vi "RTS Headers.vi"(4 "CSV Data Save Input":T1, 6 "Save Data":bool, 7 "All Data?":bool, 8 "Error In":errorcluster, 9 "RTS Config Setup Input":T3, 10 "Station":u8=1 min=1 max=8 step=1, 11 "Chamber 1 Data in":T12 {"Room PID Settings"."Room Dehumid Temperature I (*RM Dehum I1)" max=30000 step=1; "Room PID Settings"."Room Dehumid Temperature P (*RM Dehum P1)" max=30000 step=1; "Room PID Settings"."Room Cool Temperature I (*RM Cool I1)" max=30000 step=1; "Room PID Settings"."Room Cool Temperature P (*RM Cool P1)" max=30000 step=1; "Room PID Settings"."Room Heat I (*RM Heat I1)" max=30000 step=1; "Room PID Settings"."Room Heat P (*RM Heat P1)" max=30000 step=1; "Room PID Settings"."Room Humidity I (*RM Hum I1)" max=30000 step=1; "Room PID Settings"."Room Humidity P (*RM Hum P1)" max=30000 step=1; "Room PID Settings"."Room Dry I (*RM Dry I1)" max=30000 step=1; "Room PID Settings"."Room Dry P(*RM Dry P1)" max=30000 step=1; "Station 8"."Voltage (V):Element 1 Avg" format="%.3g"; "Station 8"."Voltage (V):Element 2 Avg" format="%.3g"; "Station 8"."Max Watt Hours" format="%.3g"; "Station 8"."Power Factor:Element 2" format="%.3g"; "Station 8"."Power Factor:Element 1" format="%.3g"; "Station 8"."Apparent Power (VA):Element 2" format="%.3g"; "Station 8"."Apparent Power (VA):Element 1" format="%.3g"; "Station 8"."Frequency (Hz):Element 1" format="%.3g"; "Station 8"."Time:Element 1" format="%.3g"; "Station 8"."Voltage Crest Factor:Element 2" format="%.3g"; "Station 8"."Voltage Crest Factor:Element 1" format="%.3g"; "Station 8"."Voltage Harmonic (%):Element 2" format="%.3g"; "Station 8"."Voltage Harmonic (%):Element 1" format="%.3g"; "Station 8"."Current Crest Factor:Element 2" format="%.3g"; "Station 8"."Current Crest Factor:Element 1" format="%.3g"; "Station 8"."Voltage (V):Element 1" format="%.3g"; "Station 8"."Voltage (V):Element 2" format="%.3g"; "Station 8"."Watt Hours (Wh):Sigma" format="%.3f"; "Station 8"."Power (W):Sigma" format="%.3g"; "Station 8"."Current (A):Element 2" format="%.3g"; "Station 8"."Current (A):Element 1" format="%.3g"; "Station 7"."Voltage (V):Element 1 Avg" format="%.3g"; "Station 7"."Voltage (V):Element 2 Avg" format="%.3g"; "Station 7"."Max Watt Hours" format="%.3g"; "Station 7"."Power Factor:Element 2" format="%.3g"; "Station 7"."Power Factor:Element 1" format="%.3g"; "Station 7"."Apparent Power (VA):Element 2" format="%.3g"; "Station 7"."Apparent Power (VA):Element 1" format="%.3g"; "Station 7"."Frequency (Hz):Element 1" format="%.3g"; "Station 7"."Time:Element 1" format="%.3g"; "Station 7"."Voltage Crest Factor:Element 2" format="%.3g"; "Station 7"."Voltage Crest Factor:Element 1" format="%.3g"; "Station 7"."Voltage Harmonic (%):Element 2" format="%.3g"; "Station 7"."Voltage Harmonic (%):Element 1" format="%.3g"; "Station 7"."Current Crest Factor:Element 2" format="%.3g"; "Station 7"."Current Crest Factor:Element 1" format="%.3g"; "Station 7"."Voltage (V):Element 1" format="%.3g"; "Station 7"."Voltage (V):Element 2" format="%.3g"; "Station 7"."Watt Hours (Wh):Sigma" format="%.3f"; "Station 7"."Power (W):Sigma" format="%.3g"; "Station 7"."Current (A):Element 2" format="%.3g"; "Station 7"."Current (A):Element 1" format="%.3g"; "Station 6"."Voltage (V):Element 1 Avg" format="%.3g"; "Station 6"."Voltage (V):Element 2 Avg" format="%.3g"; "Station 6"."Max Watt Hours" format="%.3g"; "Station 6"."Power Factor:Element 2" format="%.3g"; "Station 6"."Power Factor:Element 1" format="%.3g"; "Station 6"."Apparent Power (VA):Element 2" format="%.3g"; "Station 6"."Apparent Power (VA):Element 1" format="%.3g"; "Station 6"."Frequency (Hz):Element 1" format="%.3g"; "Station 6"."Time:Element 1" format="%.3g"; "Station 6"."Voltage Crest Factor:Element 2" format="%.3g"; "Station 6"."Voltage Crest Factor:Element 1" format="%.3g"; "Station 6"."Voltage Harmonic (%):Element 2" format="%.3g"; "Station 6"."Voltage Harmonic (%):Element 1" format="%.3g"; "Station 6"."Current Crest Factor:Element 2" format="%.3g"; "Station 6"."Current Crest Factor:Element 1" format="%.3g"; "Station 6"."Voltage (V):Element 1" format="%.3g"; "Station 6"."Voltage (V):Element 2" format="%.3g"; "Station 6"."Watt Hours (Wh):Sigma" format="%.3f"; "Station 6"."Power (W):Sigma" format="%.3g"; "Station 6"."Current (A):Element 2" format="%.3g"; "Station 6"."Current (A):Element 1" format="%.3g"; "Station 5"."Voltage (V):Element 1 Avg" format="%.3g"; "Station 5"."Voltage (V):Element 2 Avg" format="%.3g"; "Station 5"."Max Watt Hours" format="%.3g"; "Station 5"."Power Factor:Element 2" format="%.3g"; "Station 5"."Power Factor:Element 1" format="%.3g"; "Station 5"."Apparent Power (VA):Element 2" format="%.3g"; "Station 5"."Apparent Power (VA):Element 1" format="%.3g"; "Station 5"."Frequency (Hz):Element 1" format="%.3g"; "Station 5"."Time:Element 1" format="%.3g"; "Station 5"."Voltage Crest Factor:Element 2" format="%.3g"; "Station 5"."Voltage Crest Factor:Element 1" format="%.3g"; "Station 5"."Voltage Harmonic (%):Element 2" format="%.3g"; "Station 5"."Voltage Harmonic (%):Element 1" format="%.3g"; "Station 5"."Current Crest Factor:Element 2" format="%.3g"; "Station 5"."Current Crest Factor:Element 1" format="%.3g"; "Station 5"."Voltage (V):Element 1" format="%.3g"; "Station 5"."Voltage (V):Element 2" format="%.3g"; "Station 5"."Watt Hours (Wh):Sigma" format="%.3f"; "Station 5"."Power (W):Sigma" format="%.3g"; "Station 5"."Current (A):Element 2" format="%.3g"; "Station 5"."Current (A):Element 1" format="%.3g"; "Station 4"."Voltage (V):Element 1 Avg" format="%.3g"; "Station 4"."Voltage (V):Element 2 Avg" format="%.3g"; "Station 4"."Max Watt Hours" format="%.3g"; "Station 4"."Power Factor:Element 2" format="%.3g"; "Station 4"."Power Factor:Element 1" format="%.3g"; "Station 4"."Apparent Power (VA):Element 2" format="%.3g"; "Station 4"."Apparent Power (VA):Element 1" format="%.3g"; "Station 4"."Frequency (Hz):Element 1" format="%.3g"; "Station 4"."Time:Element 1" format="%.3g"; "Station 4"."Voltage Crest Factor:Element 2" format="%.3g"; "Station 4"."Voltage Crest Factor:Element 1" format="%.3g"; "Station 4"."Voltage Harmonic (%):Element 2" format="%.3g"; "Station 4"."Voltage Harmonic (%):Element 1" format="%.3g"; "Station 4"."Current Crest Factor:Element 2" format="%.3g"; "Station 4"."Current Crest Factor:Element 1" format="%.3g"; "Station 4"."Voltage (V):Element 1" format="%.3g"; "Station 4"."Voltage (V):Element 2" format="%.3g"; "Station 4"."Watt Hours (Wh):Sigma" format="%.3f"; "Station 4"."Power (W):Sigma" format="%.3g"; "Station 4"."Current (A):Element 2" format="%.3g"; "Station 4"."Current (A):Element 1" format="%.3g"; "Station 3"."Voltage (V):Element 1 Avg" format="%.3g"; "Station 3"."Voltage (V):Element 2 Avg" format="%.3g"; "Station 3"."Max Watt Hours" format="%.3g"; "Station 3"."Power Factor:Element 2" format="%.3g"; "Station 3"."Power Factor:Element 1" format="%.3g"; "Station 3"."Apparent Power (VA):Element 2" format="%.3g"; "Station 3"."Apparent Power (VA):Element 1" format="%.3g"; "Station 3"."Frequency (Hz):Element 1" format="%.3g"; "Station 3"."Time:Element 1" format="%.3g"; "Station 3"."Voltage Crest Factor:Element 2" format="%.3g"; "Station 3"."Voltage Crest Factor:Element 1" format="%.3g"; "Station 3"."Voltage Harmonic (%):Element 2" format="%.3g"; "Station 3"."Voltage Harmonic (%):Element 1" format="%.3g"; "Station 3"."Current Crest Factor:Element 2" format="%.3g"; "Station 3"."Current Crest Factor:Element 1" format="%.3g"; "Station 3"."Voltage (V):Element 1" format="%.3g"; "Station 3"."Voltage (V):Element 2" format="%.3g"; "Station 3"."Watt Hours (Wh):Sigma" format="%.3f"; "Station 3"."Power (W):Sigma" format="%.3g"; "Station 3"."Current (A):Element 2" format="%.3g"; "Station 3"."Current (A):Element 1" format="%.3g"; "Station 2"."Voltage (V):Element 1 Avg" format="%.3g"; "Station 2"."Voltage (V):Element 2 Avg" format="%.3g"; "Station 2"."Max Watt Hours" format="%.3g"; "Station 2"."Power Factor:Element 2" format="%.3g"; "Station 2"."Power Factor:Element 1" format="%.3g"; "Station 2"."Apparent Power (VA):Element 2" format="%.3g"; "Station 2"."Apparent Power (VA):Element 1" format="%.3g"; "Station 2"."Frequency (Hz):Element 1" format="%.3g"; "Station 2"."Time:Element 1" format="%.3g"; "Station 2"."Voltage Crest Factor:Element 2" format="%.3g"; "Station 2"."Voltage Crest Factor:Element 1" format="%.3g"; "Station 2"."Voltage Harmonic (%):Element 2" format="%.3g"; "Station 2"."Voltage Harmonic (%):Element 1" format="%.3g"; "Station 2"."Current Crest Factor:Element 2" format="%.3g"; "Station 2"."Current Crest Factor:Element 1" format="%.3g"; "Station 2"."Voltage (V):Element 1" format="%.3g"; "Station 2"."Voltage (V):Element 2" format="%.3g"; "Station 2"."Watt Hours (Wh):Sigma" format="%.3f"; "Station 2"."Power (W):Sigma" format="%.3g"; "Station 2"."Current (A):Element 2" format="%.3g"; "Station 2"."Current (A):Element 1" format="%.3g"; "Station 1"."Voltage (V):Element 1 Avg" format="%.3g"; "Station 1"."Voltage (V):Element 2 Avg" format="%.3g"; "Station 1"."Max Watt Hours" format="%.3g"; "Station 1"."Power Factor:Element 2" format="%.3g"; "Station 1"."Power Factor:Element 1" format="%.3g"; "Station 1"."Apparent Power (VA):Element 2" format="%.3g"; "Station 1"."Apparent Power (VA):Element 1" format="%.3g"; "Station 1"."Frequency (Hz):Element 1" format="%.3g"; "Station 1"."Time:Element 1" format="%.3g"; "Station 1"."Voltage Crest Factor:Element 2" format="%.3g"; "Station 1"."Voltage Crest Factor:Element 1" format="%.3g"; "Station 1"."Voltage Harmonic (%):Element 2" format="%.3g"; "Station 1"."Voltage Harmonic (%):Element 1" format="%.3g"; "Station 1"."Current Crest Factor:Element 2" format="%.3g"; "Station 1"."Current Crest Factor:Element 1" format="%.3g"; "Station 1"."Voltage (V):Element 1" format="%.3g"; "Station 1"."Voltage (V):Element 2" format="%.3g"; "Station 1"."Watt Hours (Wh):Sigma" format="%.3f"; "Station 1"."Power (W):Sigma" format="%.3g"; "Station 1"."Current (A):Element 2" format="%.3g"; "Station 1"."Current (A):Element 1" format="%.3g"}) -> (0 "Error Out":errorcluster, 2 "Custom Saved Titles":string[][](array[string]), 3 "All Data w/ Headers":string[][](array[string]))   [LabVIEW 2016]
uses:
  Type Definitions/RTS Chamber Data.ctl
  Utility/Type Definitions/UTILITY Power Data.ctl
  Type Definitions/RTS Chamber TCs.ctl
  Type Definitions/RTS MX5 AUX Data.ctl
  Drivers/WAGO 750-881/Type Definitions/Wago Door Relays.ctl
  Drivers/WAGO 750-881/Type Definitions/Wago Contactor Settings.ctl
  Drivers/WAGO 750-881/Type Definitions/Wago Ground Leakage.ctl
  Drivers/WAGO 750-881/Type Definitions/Wago Measured Input Data.ctl
  Drivers/WAGO 750-881/Type Definitions/Wago Room Setpoint Targets.ctl
  Drivers/WAGO 750-881/Type Definitions/Wago Room PID Settings.ctl
  Drivers/WAGO 750-881/Type Definitions/Wago Room Condtions.ctl
  Type Definitions/RTS Configuration Setup.ctl
  Type Definitions/RTS Wago Config.ctl
  Type Definitions/RTS APLUS Config.ctl
  Type Definitions/RTS Yokogawa MX Config.ctl
  Type Definitions/RTS Replay Server Control.ctl
  Type Definitions/RTS Server Configuration.ctl
  Type Definitions/RTS Station Settions TCP Comms.ctl
  Type Definitions/RTS Chamber Save Status.ctl
  Type Definitions/RTS Test Pattern.ctl
  Type Definitions/RTS TDMS Filename Locations.ctl
  Type Definitions/RTS Save References.ctl
panel:
  # "APLUS"
  # "MX100"
  # "Wago Controller"
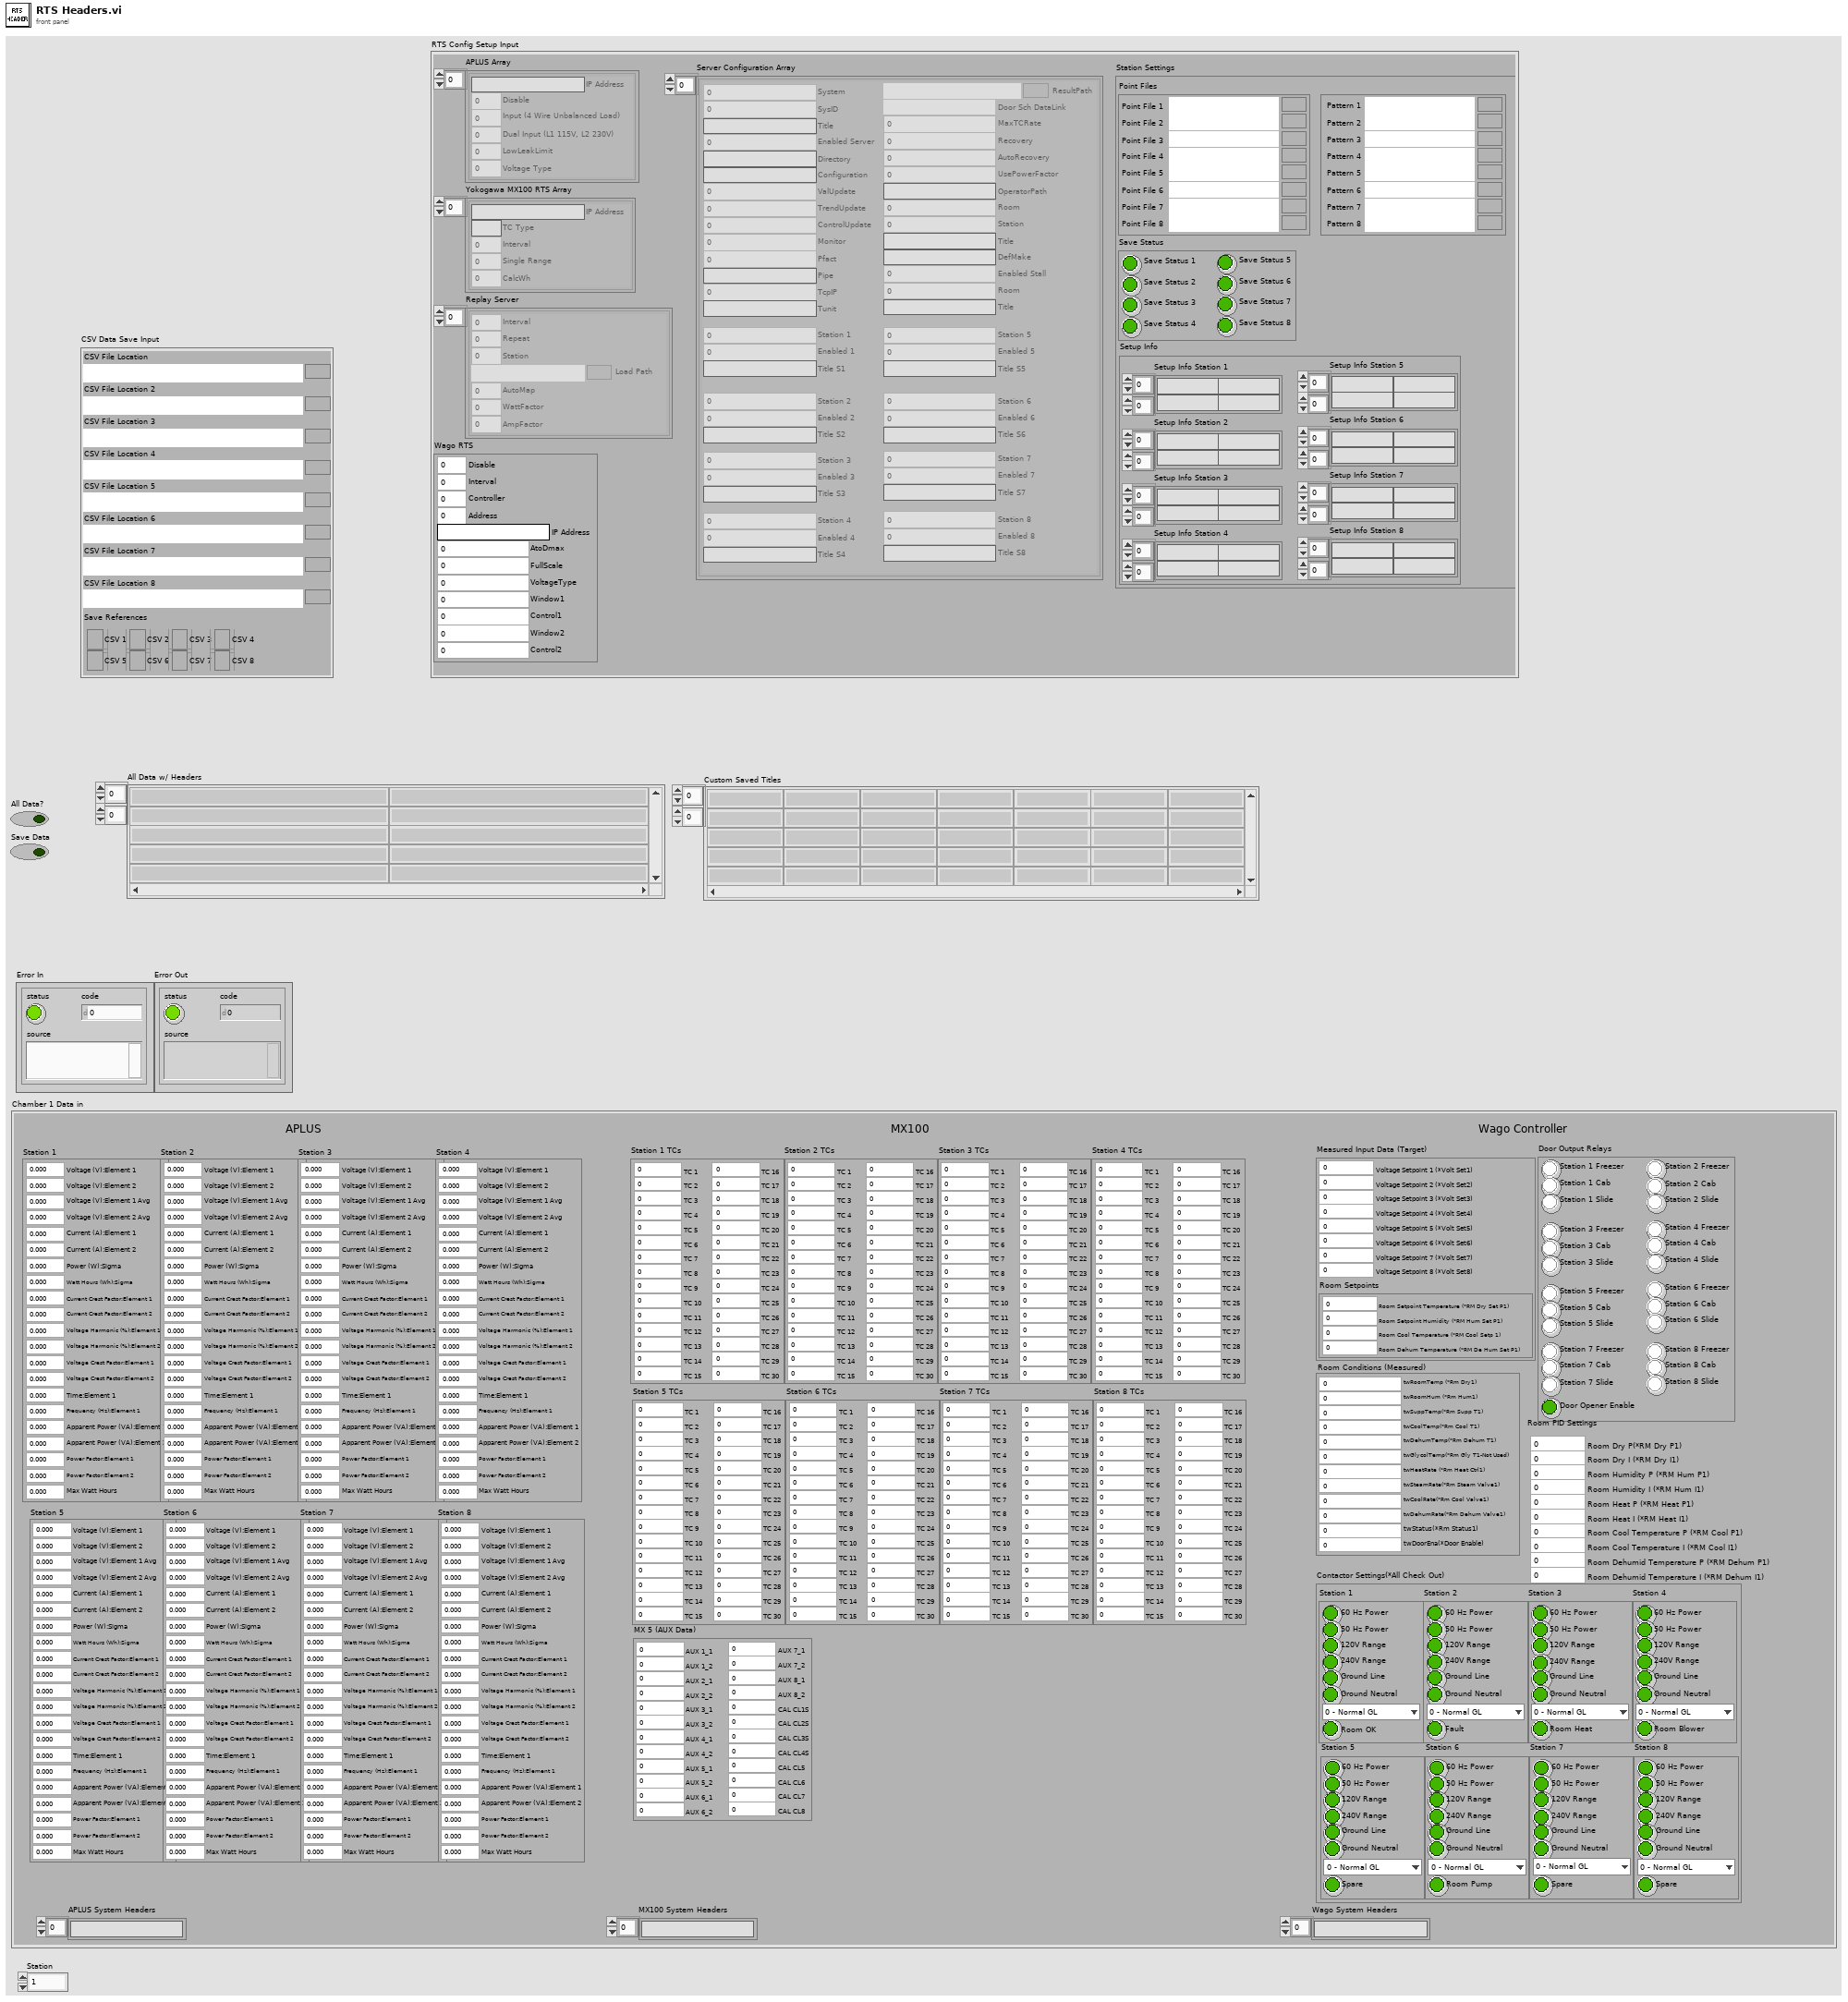
[diagram p1: front panel]
types:
  T1 = typedef "RTS TDMS Filename Locations.ctl" = cluster{"CSV File Location":path, "CSV File Location 2":path, "CSV File Location 3":path, "CSV File Location 4":path, "CSV File Location 5":path, "CSV File Location 6":path, "CSV File Location 7":path, "CSV File Location 8":path, "Save References":T2}
  T2 = typedef "RTS Save References.ctl" = cluster{"CSV 1":refnum<file>, "CSV 2":refnum<file>, "CSV 3":refnum<file>, "CSV 4":refnum<file>, "CSV 5":refnum<file>, "CSV 6":refnum<file>, "CSV 7":refnum<file>, "CSV 8":refnum<file>}
  T3 = typedef "RTS Configuration Setup.ctl" = cluster{"Wago RTS":T4, "APLUS Array":T5[], "Yokogawa MX100 RTS Array":T6[], "Replay Server":T7[], "Server Configuration Array":T8[], "Station Settings":T9}
  T4 = typedef "RTS Wago Config.ctl" = cluster{"Disable":u16, "Interval":u16, "Controller":u16, "Address":u16, "IP Address":string, "AtoDmax":u16, "FullScale":u16, "VoltageType":u16, "Window1":u16, "Control1":u16, "Window2":u16, "Control2":u16}
  T5 = typedef "RTS APLUS Config.ctl" = cluster{"Disable":u16, "IP Address":string, "Input (4 Wire Unbalanced Load)":u16, "Dual Input (L1 115V, L2 230V)":u16, "LowLeakLimit":dbl, "Voltage Type":u16}
  T6 = typedef "RTS Yokogawa MX Config.ctl" = cluster{"IP Address":string, "TC Type":string, "Interval":u16, "Single Range":u16, "CalcWh":u16}
  T7 = typedef "RTS Replay Server Control.ctl" = cluster{"Interval":i16, "Repeat":u16, "Station":u16, "Load Path":path, "AutoMap":u16, "WattFactor":dbl, "AmpFactor":dbl}
  T8 = typedef "RTS Server Configuration.ctl" = cluster{"System":u16, "SysID":u16, "Title":string, "Enabled Server":u16, "Directory":string, "Configuration":string, "ValUpdate":u16, "TrendUpdate":u16, "ControlUpdate":u16, "Monitor":u16, "Pfact":u16, "Pipe":string, "TcpIP":u16, "Tunit":string, "ResultPath":path, "Door Sch DataLink":path, "MaxTCRate":u16, "Recovery":u16, "AutoRecovery":u16, "UsePowerFactor":u16, "OperatorPath":string, "Room":u16, "Station":u16, "Title":string, "DefMake":string, "Enabled Stall":u16, "Room":u16, "Title":string, "Station 1":u16, "Enabled 1":u16, "Station 2":u16, "Enabled 2":u16, "Station 3":u16, "Enabled 3":u16, "Station 4":u16, "Enabled 4":u16, "Station 5":u16, "Enabled 5":u16, "Station 6":u16, "Enabled 6":u16, "Station 7":u16, "Enabled 7":u16, "Station 8":u16, "Enabled 8":u16, "Title S1":string, "Title S2":string, "Title S3":string, "Title S5":string, "Title S6":string, "Title S7":string, "Title S8":string, "Title S4":string}
  T9 = typedef "RTS Station Settions TCP Comms.ctl" = cluster{"Point Files":cluster{"Point File 1":path, "Point File 2":path, "Point File 3":path, "Point File 4":path, "Point File 5":path, "Point File 6":path, "Point File 7":path, "Point File 8":path}, "Save Status":T10, "Setup Info":cluster{"Setup Info Station 1":string[][], "Setup Info Station 2":string[][], "Setup Info Station 3":string[][], "Setup Info Station 4":string[][], "Setup Info Station 5":string[][], "Setup Info Station 6":string[][], "Setup Info Station 7":string[][], "Setup Info Station 8":string[][]}, "Chamber Test Pattern":T11}
  T10 = typedef "RTS Chamber Save Status.ctl" = cluster{"Save Status 1":bool, "Save Status 2":bool, "Save Status 3":bool, "Save Status 4":bool, "Save Status 5":bool, "Save Status 6":bool, "Save Status 7":bool, "Save Status 8":bool}
  T11 = typedef "RTS Test Pattern.ctl" = cluster{" Pattern 1":path, "Pattern 2":path, "Pattern 3":path, "Pattern 4":path, "Pattern 5":path, "Pattern 6":path, "Pattern 7":path, "Pattern 8":path}
  T12 = typedef "RTS Chamber Data.ctl" = cluster{"Station 1":T13, "Station 2":T13, "Station 3":T13, "Station 4":T13, "Station 5":T13, "Station 6":T13, "Station 7":T13, "Station 8":T13, "Station 1 TCs":T14, "Station 2 TCs":T14, "Station 3 TCs":T14, "Station 4 TCs":T14, "Station 5 TCs":T14, "Station 6 TCs":T14, "Station 7 TCs":T14, "Station 8 TCs":T14, "MX 5 (AUX Data)":T15, "Door Output Relays":T16, "Contactor Settings(*All Check Out)":T17, "Measured Input Data (Target)":T19, "Room PID Settings":T21, "Room Conditions (Measured)":T22, "APLUS System Headers":string[], "MX100 System Headers":string[], "Wago System Headers":string[]}
  T13 = typedef "UTILITY Power Data.ctl" = cluster{"Current (A):Element 1":dbl, "Current (A):Element 2":dbl, "Power (W):Sigma":dbl, "Watt Hours (Wh):Sigma":dbl, "Voltage (V):Element 2":dbl, "Voltage (V):Element 1":dbl, "Current Crest Factor:Element 1":dbl, "Current Crest Factor:Element 2":dbl, "Voltage Harmonic (%):Element 1":dbl, "Voltage Harmonic (%):Element 2":dbl, "Voltage Crest Factor:Element 1":dbl, "Voltage Crest Factor:Element 2":dbl, "Time:Element 1":dbl, "Frequency (Hz):Element 1":dbl, "Apparent Power (VA):Element 1":dbl, "Apparent Power (VA):Element 2":dbl, "Power Factor:Element 1":dbl, "Power Factor:Element 2":dbl, "Max Watt Hours":dbl, "Voltage (V):Element 2 Avg":dbl, "Voltage (V):Element 1 Avg":dbl}
  T14 = typedef "RTS Chamber TCs.ctl" = cluster{"TC 1":dbl, "TC 2":dbl, "TC 3":dbl, "TC 4":dbl, "TC 5":dbl, "TC 6":dbl, "TC 7":dbl, "TC 8":dbl, "TC 9":dbl, "TC 10":dbl, "TC 11":dbl, "TC 12":dbl, "TC 13":dbl, "TC 14":dbl, "TC 15":dbl, "TC 16":dbl, "TC 17":dbl, "TC 18":dbl, "TC 19":dbl, "TC 20":dbl, "TC 21":dbl, "TC 22":dbl, "TC 23":dbl, "TC 24":dbl, "TC 25":dbl, "TC 26":dbl, "TC 27":dbl, "TC 28":dbl, "TC 29":dbl, "TC 30":dbl}
  T15 = typedef "RTS MX5 AUX Data.ctl" = cluster{"AUX 1_1":dbl, "AUX 1_2":dbl, "AUX 2_1":dbl, "AUX 2_2":dbl, "AUX 3_1":dbl, "AUX 3_2":dbl, "AUX 4_1":dbl, "AUX 4_2":dbl, "AUX 5_1":dbl, "AUX 5_2":dbl, "AUX 6_1":dbl, "AUX 6_2":dbl, "AUX 7_1":dbl, "AUX 7_2":dbl, "AUX 8_1":dbl, "AUX 8_2":dbl, "CAL CL1S":dbl, "CAL CL2S":dbl, "CAL CL3S":dbl, "CAL CL4S":dbl, "CAL CL5":dbl, "CAL CL6":dbl, "CAL CL7":dbl, "CAL CL8":dbl}
  T16 = typedef "Wago Door Relays.ctl" = cluster{"Station 1 Freezer":bool, "Station 1 Cab":bool, "Station 1 Slide":bool, "Station 2 Freezer":bool, "Station 2 Cab":bool, "Station 2 Slide":bool, "Station 3 Freezer":bool, "Station 3 Cab":bool, "Station 3 Slide":bool, "Station 4 Freezer":bool, "Station 4 Cab":bool, "Station 4 Slide":bool, "Station 5 Freezer":bool, "Station 5 Cab":bool, "Station 5 Slide":bool, "Station 6 Freezer":bool, "Station 6 Cab":bool, "Station 6 Slide":bool, "Station 7 Freezer":bool, "Station 7 Cab":bool, "Station 7 Slide":bool, "Station 8 Freezer":bool, "Station 8 Cab":bool, "Station 8 Slide":bool, "Door Opener Enable":bool}
  T17 = typedef "Wago Contactor Settings.ctl" = cluster{"Station 1":cluster{"60 Hz Power":bool, "50 Hz Power":bool, "120V Range":bool, "240V Range":bool, "Ground Line":bool, "Ground Neutral":bool, "Room OK":bool, "Ground Leakage":T18}, "Station 2":cluster{"60 Hz Power":bool, "50 Hz Power":bool, "120V Range":bool, "240V Range":bool, "Ground Line":bool, "Ground Neutral":bool, "Fault":bool, "Ground Leakage":T18}, "Station 3":cluster{"60 Hz Power":bool, "50 Hz Power":bool, "120V Range":bool, "240V Range":bool, "Ground Line":bool, "Ground Neutral":bool, "Room Heat":bool, "Ground Leakage":T18}, "Station 4":cluster{"60 Hz Power":bool, "50 Hz Power":bool, "120V Range":bool, "240V Range":bool, "Ground Line":bool, "Ground Neutral":bool, "Room Blower":bool, "Ground Leakage":T18}, "Station 5":cluster{"60 Hz Power":bool, "50 Hz Power":bool, "120V Range":bool, "240V Range":bool, "Ground Line":bool, "Ground Neutral":bool, "Spare":bool, "Ground Leakage":T18}, "Station 6":cluster{"60 Hz Power":bool, "50 Hz Power":bool, "120V Range":bool, "240V Range":bool, "Ground Line":bool, "Ground Neutral":bool, "Room Pump":bool, "Ground Leakage":T18}, "Station 7":cluster{"60 Hz Power":bool, "50 Hz Power":bool, "120V Range":bool, "240V Range":bool, "Ground Line":bool, "Ground Neutral":bool, "Spare":bool, "Ground Leakage":T18}, "Station 8":cluster{"60 Hz Power":bool, "50 Hz Power":bool, "120V Range":bool, "240V Range":bool, "Ground Line":bool, "Ground Neutral":bool, "Spare":bool, "Ground Leakage":T18}}
  T18 = typedef "Wago Ground Leakage.ctl" = enum16{"0 - Normal GL", "1 - Measure GL"}
  T19 = typedef "Wago Measured Input Data.ctl" = cluster{"Voltage Setpoint 1 (*Volt Set1)":dbl, "Voltage Setpoint 2 (*Volt Set2)":dbl, "Voltage Setpoint 3 (*Volt Set3)":dbl, "Voltage Setpoint 4 (*Volt Set4)":dbl, "Voltage Setpoint 5 (*Volt Set5)":dbl, "Voltage Setpoint 6 (*Volt Set6)":dbl, "Voltage Setpoint 7 (*Volt Set7)":dbl, "Voltage Setpoint 8 (*Volt Set8)":dbl, "Room Setpoints":T20}
  T20 = typedef "Wago Room Setpoint Targets.ctl" = cluster{"Room Setpoint Temperature (*RM Dry Set P1)":dbl, "Room Setpoint Humidity (*RM Hum Set P1)":dbl, "Room Cool Temperature (*RM Cool Setp 1)":dbl, "Room Dehum Temperature (*RM De Hum Set P1)":dbl}
  T21 = typedef "Wago Room PID Settings.ctl" = cluster{"Room Dry P(*RM Dry P1)":u16, "Room Dry I (*RM Dry I1)":u16, "Room Humidity P (*RM Hum P1)":u16, "Room Humidity I (*RM Hum I1)":u16, "Room Heat P (*RM Heat P1)":u16, "Room Heat I (*RM Heat I1)":u16, "Room Cool Temperature P (*RM Cool P1)":u16, "Room Cool Temperature I (*RM Cool I1)":u16, "Room Dehumid Temperature P (*RM Dehum P1)":u16, "Room Dehumid Temperature I (*RM Dehum I1)":u16}
  T22 = typedef "Wago Room Condtions.ctl" = cluster{"twDoorEna(*Door Enable)":u16, "twStatus(*Rm Status1)":u16, "twRoomTemp (*Rm Dry1)":dbl, "twRoomHum (*Rm Hum1)":dbl, "twSuppTemp(*Rm Supp T1)":dbl, "twCoolTemp(*Rm Cool T1)":dbl, "twDehumTemp(*Rm Dehum T1)":dbl, "twGlycolTemp(*Rm Gly T1-Not Used)":dbl, "twDehumRate(*Rm Dehum Valve1)":dbl, "twCoolRate(*Rm Cool Valve1)":dbl, "twSteamRate(*Rm Steam Valve1)":dbl, "twHeatRate (*Rm Heat Ctrl1)":dbl}
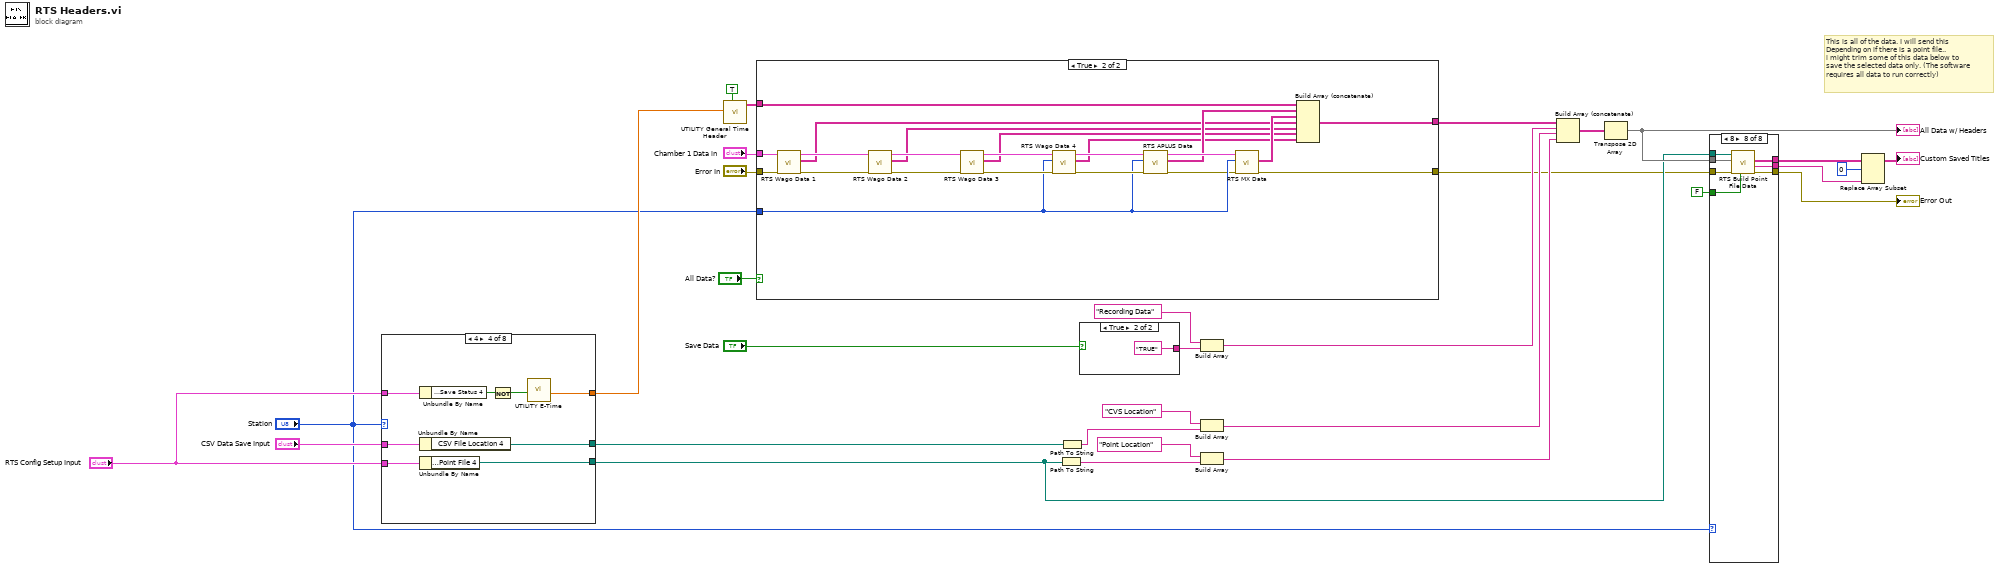
[diagram p0: block diagram]
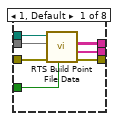
[diagram p2: hidden frame]
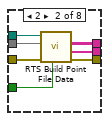
[diagram p3: hidden frame]
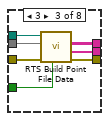
[diagram p4: hidden frame]
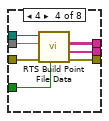
[diagram p5: hidden frame]
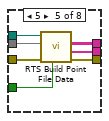
[diagram p6: hidden frame]
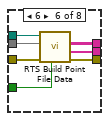
[diagram p7: hidden frame]
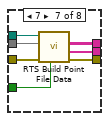
[diagram p8: hidden frame]
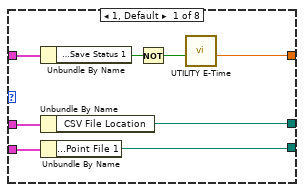
[diagram p9: hidden frame]
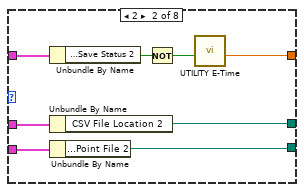
[diagram p10: hidden frame]
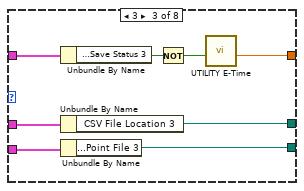
[diagram p11: hidden frame]
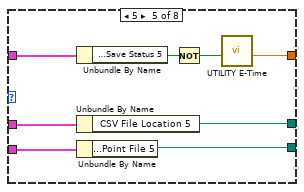
[diagram p12: hidden frame]
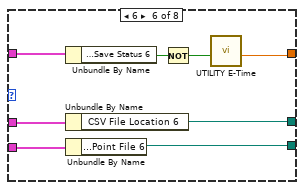
[diagram p13: hidden frame]
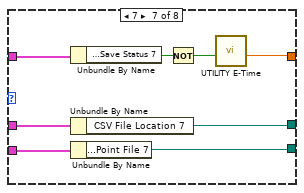
[diagram p14: hidden frame]
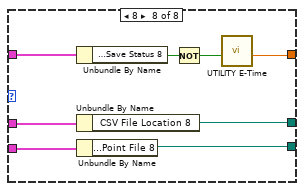
[diagram p15: hidden frame]
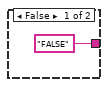
[diagram p16: hidden frame]
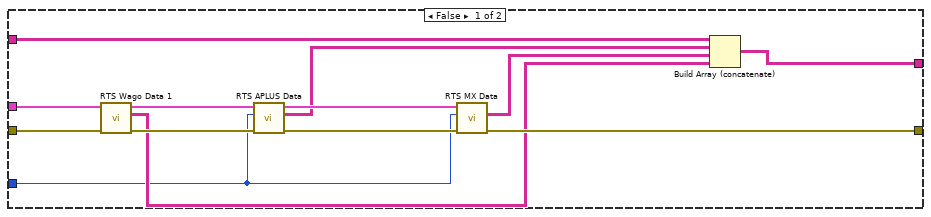
[diagram p17: hidden frame]
diagram:
  # "This is all of the data. I will send this\nDepending on if there is a point file..\ni might trim some of this data below to\nsave the selected data only. (The software \nrequires all data to run correctly)"
  n1 = case shown="4" "Station" {
    tunnel: "CSV Data Save Input" -> [w39 w47 w55 w63 w71 w79 w87 w95]
    tunnel: "RTS Config Setup Input" -> [w38 w46 w54 w62 w70 w78 w86 w94]
    tunnel: [w37 w45 w53 w61 w69 w77 w85 w93] -> w19
    tunnel: [w36 w44 w52 w60 w68 w76 w84 w92] -> w9
    tunnel: "RTS Config Setup Input" -> [w33 w41 w49 w57 w65 w73 w81 w89]
    tunnel: [w32 w40 w48 w56 w64 w72 w80 w88] -> w11
    frame 1, Default {
      n2 = Unbundle By Name(w33) -> ("Station Settings.Save Status.Save Status 1"=w34:bool)
      n3 = Unbundle By Name(w39) -> ("CSV File Location"=w37:path)
      n4 = Unbundle By Name(w38) -> ("Station Settings.Point Files.Point File 1"=w36:path)
      n5 = Not(x=w34) -> (.not. x?=w35:bool)
      n6 = call "UTILITY E-Time.vi"("Reset"=w35) -> ("Elapsed Time (sec)"=w32:dbl)  [unwired: 8 in, 2 out]
    }
    frame 2 {
      n7 = Unbundle By Name(w41) -> ("Station Settings.Save Status.Save Status 2"=w43:bool)
      n8 = Unbundle By Name(w47) -> ("CSV File Location 2"=w45:path)
      n9 = Unbundle By Name(w46) -> ("Station Settings.Point Files.Point File 2"=w44:path)
      n10 = Not(x=w43) -> (.not. x?=w42:bool)
      n11 = call "UTILITY E-Time.vi"("Reset"=w42) -> ("Elapsed Time (sec)"=w40:dbl)  [unwired: 8 in, 2 out]
    }
    frame 3 {
      n12 = Unbundle By Name(w49) -> ("Station Settings.Save Status.Save Status 3"=w51:bool)
      n13 = Unbundle By Name(w55) -> ("CSV File Location 3"=w53:path)
      n14 = Unbundle By Name(w54) -> ("Station Settings.Point Files.Point File 3"=w52:path)
      n15 = Not(x=w51) -> (.not. x?=w50:bool)
      n16 = call "UTILITY E-Time.vi"("Reset"=w50) -> ("Elapsed Time (sec)"=w48:dbl)  [unwired: 8 in, 2 out]
    }
    frame 4 {
      n17 = Unbundle By Name(w57) -> ("Station Settings.Save Status.Save Status 4"=w59:bool)
      n18 = Unbundle By Name(w63) -> ("CSV File Location 4"=w61:path)
      n19 = Unbundle By Name(w62) -> ("Station Settings.Point Files.Point File 4"=w60:path)
      n20 = Not(x=w59) -> (.not. x?=w58:bool)
      n21 = call "UTILITY E-Time.vi"("Reset"=w58) -> ("Elapsed Time (sec)"=w56:dbl)  [unwired: 8 in, 2 out]
    }
    frame 5 {
      n22 = Unbundle By Name(w65) -> ("Station Settings.Save Status.Save Status 5"=w67:bool)
      n23 = Unbundle By Name(w71) -> ("CSV File Location 5"=w69:path)
      n24 = Unbundle By Name(w70) -> ("Station Settings.Point Files.Point File 5"=w68:path)
      n25 = Not(x=w67) -> (.not. x?=w66:bool)
      n26 = call "UTILITY E-Time.vi"("Reset"=w66) -> ("Elapsed Time (sec)"=w64:dbl)  [unwired: 8 in, 2 out]
    }
    frame 6 {
      n27 = Unbundle By Name(w73) -> ("Station Settings.Save Status.Save Status 6"=w75:bool)
      n28 = Unbundle By Name(w79) -> ("CSV File Location 6"=w77:path)
      n29 = Unbundle By Name(w78) -> ("Station Settings.Point Files.Point File 6"=w76:path)
      n30 = Not(x=w75) -> (.not. x?=w74:bool)
      n31 = call "UTILITY E-Time.vi"("Reset"=w74) -> ("Elapsed Time (sec)"=w72:dbl)  [unwired: 8 in, 2 out]
    }
    frame 7 {
      n32 = Unbundle By Name(w81) -> ("Station Settings.Save Status.Save Status 7"=w83:bool)
      n33 = Unbundle By Name(w87) -> ("CSV File Location 7"=w85:path)
      n34 = Unbundle By Name(w86) -> ("Station Settings.Point Files.Point File 7"=w84:path)
      n35 = Not(x=w83) -> (.not. x?=w82:bool)
      n36 = call "UTILITY E-Time.vi"("Reset"=w82) -> ("Elapsed Time (sec)"=w80:dbl)  [unwired: 8 in, 2 out]
    }
    frame 8 {
      n37 = Unbundle By Name(w89) -> ("Station Settings.Save Status.Save Status 8"=w91:bool)
      n38 = Unbundle By Name(w95) -> ("CSV File Location 8"=w93:path)
      n39 = Unbundle By Name(w94) -> ("Station Settings.Point Files.Point File 8"=w92:path)
      n40 = Not(x=w91) -> (.not. x?=w90:bool)
      n41 = call "UTILITY E-Time.vi"("Reset"=w90) -> ("Elapsed Time (sec)"=w88:dbl)  [unwired: 8 in, 2 out]
    }
  }
  n42 = call "UTILITY General Time Header.vi"("Add Elapsed Time (hrs)"=TRUE, "Elapsed Time"=w11) -> ("Total Array"=w13:string[][])  [unwired: 8 in, 1 out]
  n43 = case shown="True" "All Data?" {
    tunnel: "Chamber 1 Data in" -> [w104 w122]
    tunnel: "Station" -> [w96 w120]
    tunnel: w13 -> [w101 w118]
    tunnel: [w97 w111] -> w23
    tunnel: "Error In" -> [w108 w110]
    tunnel: [w105 w109] -> w8
    frame False {
      n44 = call "RTS Wago Data 1.vi"("Error In"=w108, "Chamber 1 Data in"=w104) -> ("Error Out"=w107:errorcluster, "Data 1 Output"=w98:string[][], "Chamber 1 Data Out"=w103:T12)  [unwired: 6 in, 1 out]
      n45 = call "RTS APLUS Data.vi"("Error In"=w107, "Station"=w96, "Chamber 1 Data Out"=w103) -> ("Error Out"=w106:errorcluster, "Data"=w100:string[][], "Chamber 1 Data"=w102:T12)  [unwired: 5 in, 1 out]
      n46 = call "RTS MX Data.vi"("Error In"=w106, "Station"=w96, "Chamber 1 Data in"=w102) -> ("Error Out"=w105:errorcluster, "Data MX"=w99:string[][])  [unwired: 5 in, 2 out]
      n47 = Build Array (concatenate)(w101, w100, w99, w98) -> (w97:string[][])
    }
    frame True {
      n48 = call "RTS Wago Data 1.vi"("Error In"=w110, "Chamber 1 Data in"=w122) -> ("Error Out"=w129:errorcluster, "Data 1 Output"=w115:string[][], "Chamber 1 Data Out"=w130:T12)  [unwired: 6 in, 1 out]
      n49 = call "RTS Wago Data 2.vi"("Error In"=w129, "Chamber 1 Data in"=w130) -> ("Error Out"=w127:errorcluster, "Data 2"=w114:string[][], "Chamber 1 Data Out"=w128:T12)  [unwired: 6 in, 1 out]
      n50 = call "RTS Wago Data 3.vi"("Error In"=w127, "Chamber 1 Data in"=w128) -> ("Error Out"=w125:errorcluster, "Data 3"=w113:string[][], "Chamber 1 Data Out"=w126:T12)  [unwired: 6 in, 1 out]
      n51 = call "RTS Wago Data 4.vi"("Error In"=w125, "Station"=w120, "Chamber 1 Data in"=w126) -> ("Error Out"=w123:errorcluster, "Data 4"=w112:string[][], "Chamber 1 Data Out"=w124:T12)  [unwired: 5 in, 1 out]
      n52 = call "RTS APLUS Data.vi"("Error In"=w123, "Station"=w120, "Chamber 1 Data Out"=w124) -> ("Error Out"=w119:errorcluster, "Data"=w117:string[][], "Chamber 1 Data"=w121:T12)  [unwired: 5 in, 1 out]
      n53 = call "RTS MX Data.vi"("Error In"=w119, "Station"=w120, "Chamber 1 Data in"=w121) -> ("Error Out"=w109:errorcluster, "Data MX"=w116:string[][])  [unwired: 5 in, 2 out]
      n54 = Build Array (concatenate)(w118, w117, w116, w115, w114, w113, w112) -> (w111:string[][])
    }
  }
  n55 = Path To String(path=w9) -> (string=w18:string)
  n56 = Path To String(path=w19) -> (string=w17:string)
  n57 = case shown="True" "Save Data" {
    tunnel: ["FALSE" "TRUE"] -> w27
    frame False {
    }
    frame True {
    }
  }
  n58 = Build Array("Recording Data" ("String"), w27) -> (w25:string[])
  n59 = Build Array("CVS Location" ("String"), w17) -> (w16:string[])
  n60 = Build Array("Point Location" ("String"), w18) -> (w15:string[])
  n61 = Build Array (concatenate)(w23, w25, w16, w15) -> (w24:string[][])
  n62 = Transpose 2D Array(2D array=w24) -> (transposed array=w10:string[][])
  "All Data w/ Headers" <- w10
  n63 = case shown="8" "Station" {
    tunnel: w10 -> [w139 w143 w150 w157 w164 w171 w178 w185]
    tunnel: w9 -> [w138 w144 w151 w158 w165 w172 w179 w186]
    tunnel: w8 -> [w137 w146 w153 w160 w167 w174 w181 w188]
    tunnel: [w136 w145 w152 w159 w166 w173 w180 w187] -> w7
    tunnel: [w135 w142 w149 w156 w163 w170 w177 w184] -> w6
    tunnel: [w134 w141 w148 w155 w162 w169 w176 w183] -> w5
    tunnel: FALSE ("Disable System Time Filter") -> [w133 w140 w147 w154 w161 w168 w175 w182]
    frame 1, Default {
      n64 = call "RTS Build Point File Data.vi"("Disable System Time Filter"=w133, "Error In"=w137, "Full List Box Data"=w139, "Point File Location"=w138) -> ("Error Out"=w136:errorcluster, "Custom Titles"=w134:string[], "Custom Listbox Data"=w135:string[][])  [unwired: 4 in, 1 out]
    }
    frame 2 {
      n65 = call "RTS Build Point File Data.vi"("Disable System Time Filter"=w140, "Error In"=w146, "Full List Box Data"=w143, "Point File Location"=w144) -> ("Error Out"=w145:errorcluster, "Custom Titles"=w141:string[], "Custom Listbox Data"=w142:string[][])  [unwired: 4 in, 1 out]
    }
    frame 3 {
      n66 = call "RTS Build Point File Data.vi"("Disable System Time Filter"=w147, "Error In"=w153, "Full List Box Data"=w150, "Point File Location"=w151) -> ("Error Out"=w152:errorcluster, "Custom Titles"=w148:string[], "Custom Listbox Data"=w149:string[][])  [unwired: 4 in, 1 out]
    }
    frame 4 {
      n67 = call "RTS Build Point File Data.vi"("Disable System Time Filter"=w154, "Error In"=w160, "Full List Box Data"=w157, "Point File Location"=w158) -> ("Error Out"=w159:errorcluster, "Custom Titles"=w155:string[], "Custom Listbox Data"=w156:string[][])  [unwired: 4 in, 1 out]
    }
    frame 5 {
      n68 = call "RTS Build Point File Data.vi"("Disable System Time Filter"=w161, "Error In"=w167, "Full List Box Data"=w164, "Point File Location"=w165) -> ("Error Out"=w166:errorcluster, "Custom Titles"=w162:string[], "Custom Listbox Data"=w163:string[][])  [unwired: 4 in, 1 out]
    }
    frame 6 {
      n69 = call "RTS Build Point File Data.vi"("Disable System Time Filter"=w168, "Error In"=w174, "Full List Box Data"=w171, "Point File Location"=w172) -> ("Error Out"=w173:errorcluster, "Custom Titles"=w169:string[], "Custom Listbox Data"=w170:string[][])  [unwired: 4 in, 1 out]
    }
    frame 7 {
      n70 = call "RTS Build Point File Data.vi"("Disable System Time Filter"=w175, "Error In"=w181, "Full List Box Data"=w178, "Point File Location"=w179) -> ("Error Out"=w180:errorcluster, "Custom Titles"=w176:string[], "Custom Listbox Data"=w177:string[][])  [unwired: 4 in, 1 out]
    }
    frame 8 {
      n71 = call "RTS Build Point File Data.vi"("Disable System Time Filter"=w182, "Error In"=w188, "Full List Box Data"=w185, "Point File Location"=w186) -> ("Error Out"=w187:errorcluster, "Custom Titles"=w183:string[], "Custom Listbox Data"=w184:string[][])  [unwired: 4 in, 1 out]
    }
  }
  "Error Out" <- w7
  n72 = Replace Array Subset(array=w6, new element=w5, index (row)=0 ("disabled index (col)")) -> (→"Custom Saved Titles":string[][])  [unwired: 1 in]
